vi "Histogram Update.vi"(0 "Lat Hist at Trial Fraction":dbl[][](array[numeric]), 2 "Test Trial Plot Color Array IN":u32[](array[numeric]), 8 "Trial Fraction Interval":dbl) -> (14 "Hist Plot1 Trial":string, 15 "Hist Plot1 Data":dbl[](array[numeric]), 16 "Hist Plot2 Trial":string, 17 "Hist Plot2 Data":dbl[](array[numeric]), 18 "Lat Hist at Trial Fraction OUT":dbl[](array[numeric]))   [LabVIEW 2018]
uses:
  Globals/Global - Configuration Options.vi
panel:
  out "Test Trial Plot Color Array OUT":u32[](array[numeric])
  out "Test Trial":string[](array[string])
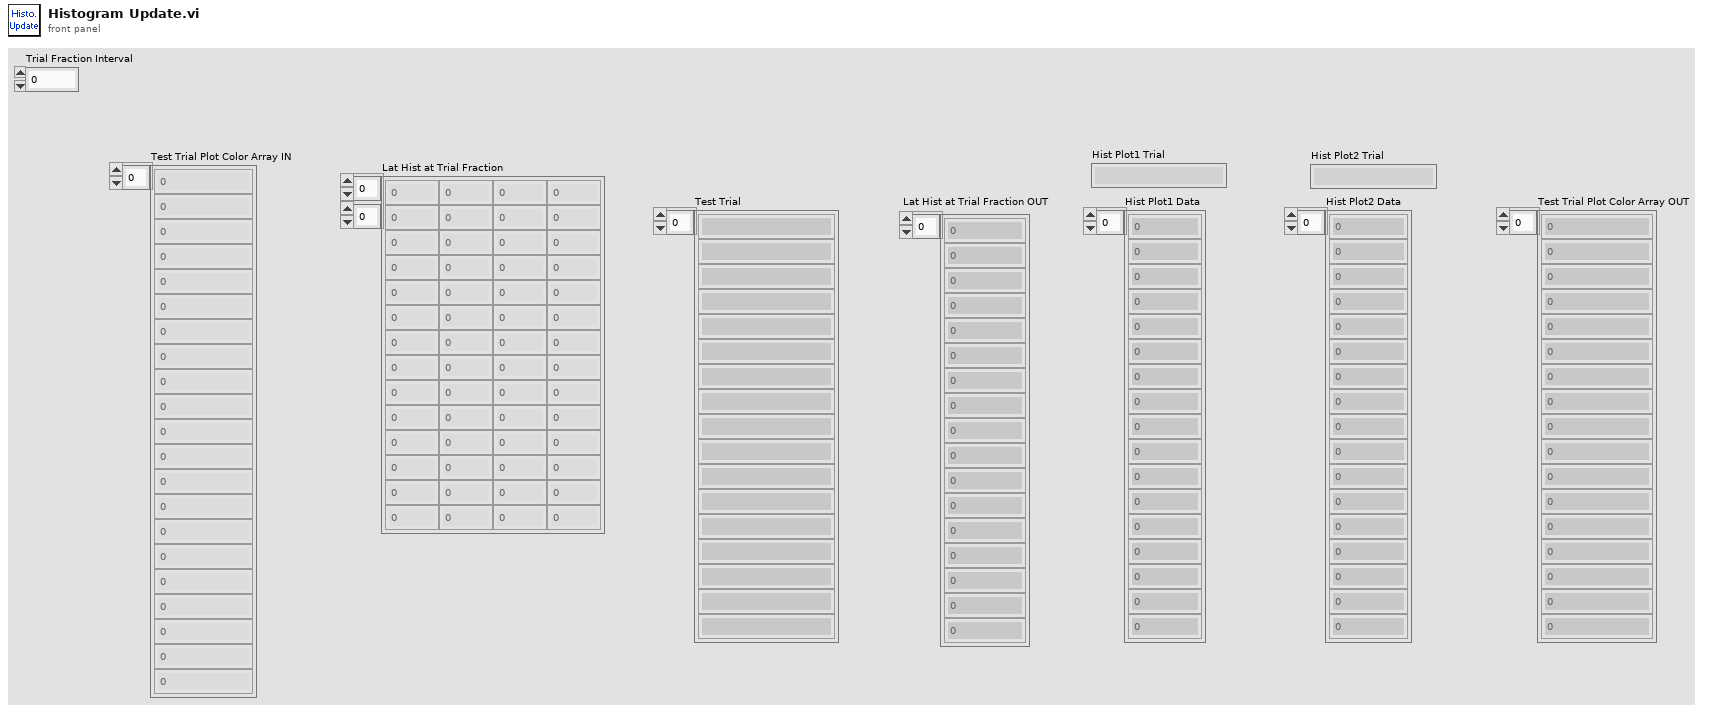
[diagram p1: front panel]
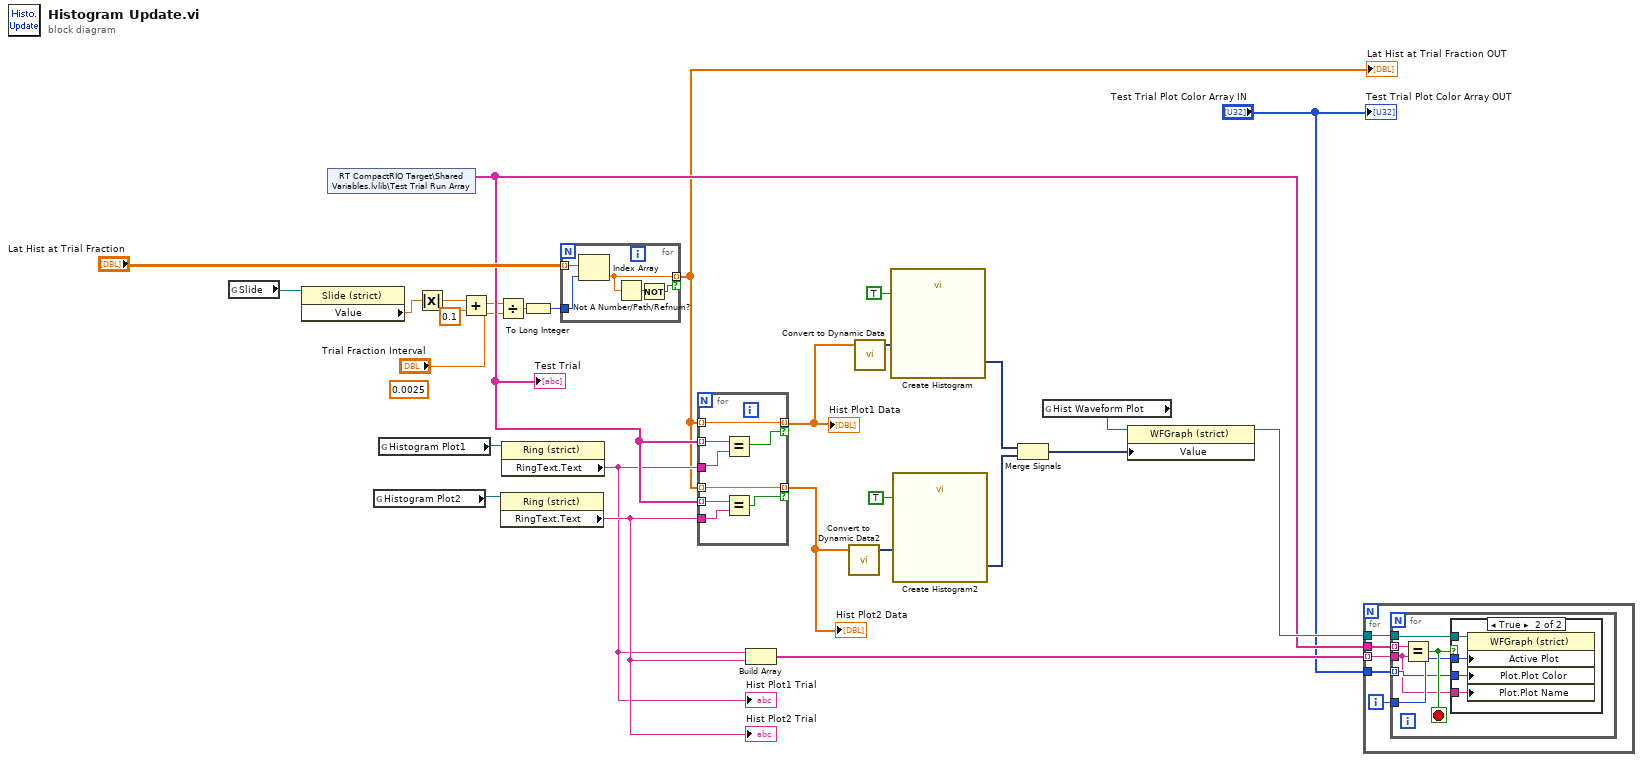
[diagram p0: block diagram]
diagram:
  (unwired) 0.0025
  n1 = global read "Global - Configuration Options.vi" "Slide"() -> (w27:refnum<vi>)
  n2 = property class="Slide (strict)"(reference=w27) -> ("Value"=w28:dbl)  [unwired: 1 in, 2 out]
  n3 = shared-variable "RT CompactRIO Target\\Shared Variables.lvlib\\Test Trial Run Array"() -> (w22:string[])  [unwired: 1 in, 1 out]
  "Test Trial" <- w22
  n4 = global read "Global - Configuration Options.vi" "Histogram Plot2"() -> (w16:refnum<vi>)
  n5 = global read "Global - Configuration Options.vi" "Histogram Plot1"() -> (w14:refnum<vi>)
  n6 = Absolute Value(x=w28) -> (abs(x)=w7:dbl)
  n7 = Add(x=w7, y=0.1) -> (x+y=w8:dbl)
  n8 = Divide(x=w8, y="Trial Fraction Interval") -> (x/y=w5:dbl)
  n9 = property class="Ring (strict)"(reference=w16) -> ("RingText.Text"=w20:string)  [unwired: 1 in, 2 out]
  "Hist Plot2 Trial" <- w20
  n10 = property class="Ring (strict)"(reference=w14) -> ("RingText.Text"=w19:string)  [unwired: 1 in, 2 out]
  "Hist Plot1 Trial" <- w19
  n11 = To Long Integer(number=w5) -> (32bit integer=w4:i32)
  n12 = for {
    tunnel: "Lat Hist at Trial Fraction" -> [w33] mode=indexing
    tunnel: w4 -> [w32]
    tunnel: [w31] -> w17 mode=indexing if=w29
    n13 = Index Array(array=w33, index=w32) -> (element=w31:dbl)
    n14 = Not A Number/Path/Refnum?(number/path/refnum=w31) -> (NaN/Path/Refnum?=w30:bool)
    n15 = Not(x=w30) -> (.not. x?=w29:bool)
  }
  "Lat Hist at Trial Fraction OUT" <- w17
  n16 = for {
    tunnel: w22 -> [w41] mode=indexing
    tunnel: w19 -> [w40]
    tunnel: w17 -> [w39] mode=indexing
    tunnel: [w39] -> w15 mode=indexing if=w38
    tunnel: w20 -> [w37]
    tunnel: w17 -> [w36] mode=indexing
    tunnel: [w36] -> w18 mode=indexing if=w35
    tunnel: w22 -> [w34] mode=indexing
    n17 = Equal?(x=w41, y=w40) -> (x = y?=w38:bool)
    n18 = Equal?(x=w34, y=w37) -> (x = y?=w35:bool)
  }
  "Hist Plot1 Data" <- w15
  "Hist Plot2 Data" <- w18
  n19 = Build Array(w19, w20) -> (w21:string[])
  n20 = call "Convert to Dynamic Data2"("Array"=w18) -> ("Dynamic Data Type"=w11:dynamicdata)  [unwired: 3 in]
  n21 = call "Convert to Dynamic Data"("Array"=w15) -> ("Dynamic Data Type"=w3:dynamicdata)  [unwired: 3 in]
  n22 = call "Create Histogram"("Reset"=TRUE, "Signal"=w3) -> ("Histogram"=w12:dynamicdata)  [unwired: 8 in, 1 out]
  n23 = call "Create Histogram2"("Reset"=TRUE, "Signal"=w11) -> ("Histogram"=w13:dynamicdata)  [unwired: 8 in, 1 out]
  n24 = Merge Signals(w12, w13) -> (w26:dynamicdata)
  n25 = global read "Global - Configuration Options.vi" "Hist Waveform Plot"() -> (w24:refnum<vi>)
  n26 = property class="WFGraph (strict)"(reference=w24, "Value"=w26) -> (reference out=w25:refnum<vi>)  [unwired: 1 in, 1 out]
  n27 = for {
    tunnel: w22 -> [w46]
    tunnel: w21 -> [w45] mode=indexing
    tunnel: "Test Trial Plot Color Array IN" -> [w43]
    tunnel: w25 -> [w44]
    i -> [w42]
    n28 = for {
      tunnel: w46 -> [w52] mode=indexing
      tunnel: w45 -> [w47]
      tunnel: w44 -> [w51]
      tunnel: w43 -> [w48] mode=indexing
      tunnel: w42 -> [w49]
      stop <- w50 stop-if-true
      n29 = Equal?(x=w52, y=w47) -> (x = y?=w50:bool)
      n30 = case shown="True" w50 {
        tunnel: w51 -> [_ w56]
        tunnel: w49 -> [_ w55]
        tunnel: w48 -> [_ w54]
        tunnel: w47 -> [_ w53]
        frame False {
        }
        frame True {
          n31 = property class="WFGraph (strict)"(reference=w56, "Active Plot"=w55, "Plot.Plot Color"=w54, "Plot.Plot Name"=w53) -> ()  [unwired: 1 in, 2 out]
        }
      }
    }
  }
  "Test Trial Plot Color Array OUT" <- "Test Trial Plot Color Array IN"
